vi "mul 1.vi"(1 "y":dbl, 2 "x":dbl) -> (10 "x*y":dbl)   [LabVIEW 2025]
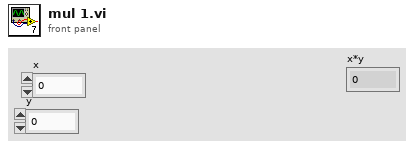
[diagram p1: front panel]
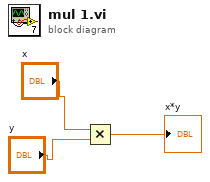
[diagram p0: block diagram]
diagram:
  n1 = Multiply(x="x", y="y") -> (x*y=→"x*y":dbl)
